vi "UEvent_ON_OFF_POWER_SOURCE.vi"(6 "USB":tag, 7 "Power ON/OFF DUT":enum16{"Power ON DUT", "Power OFF DUT"}(ring), 8 "Ext PW Vol Monitor":bool, 9 "Value":T1, 10 "Vout  - Vbat profile":enum16{"3.8VDC", "2.9VDC", "By Pass", "4.0VDC"}(ring), 11 "Refnum in":refnum<k21>) -> (1 "Battery_Voltage":dbl, 2 "DUT_Voltage":dbl, 3 "Refnum out":refnum<k21>)   [LabVIEW 2015]
uses:
  Range_Shunt_selector.ctl
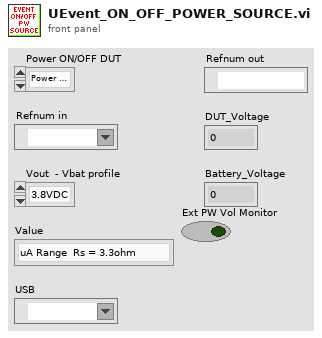
[diagram p1: front panel]
types:
  T1 = typedef "Range_Shunt_selector.ctl" = enum16{"uA Range  Rs = 3.3ohm", "mA Range Rs = 3.3ohm", "mA Range Rs = 1ohm", "mA Range Rs = 1ohm - X2"}
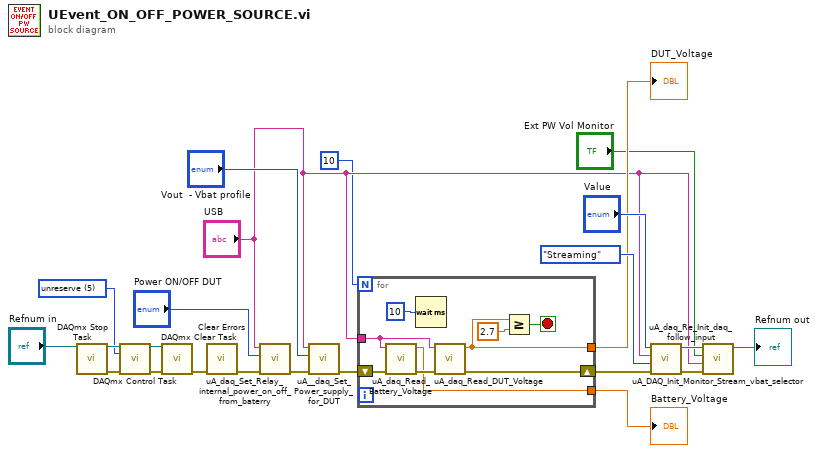
[diagram p0: block diagram]
diagram:
  w1 = 5 items=["verify"=2, "reserve"=4, "commit"=3, "unreserve"=5, "abort"=6] ("action")
  n1 = call <vilib>:"DAQmx Stop Task.vi"("task/channels in"="Refnum in") -> ("task out"=w5:refnum<k21>, "error out"=w3:errorcluster)  [unwired: 13 in]
  n2 = call <vilib>:"DAQmx Control Task.vi"("task/channels in"=w5, "action"=w1, "error in"=w3) -> ("task out"=w4:refnum<k21>, "error out"=w2:errorcluster)  [unwired: 11 in]
  n3 = call <vilib>:"DAQmx Clear Task.vi"("task in"=w4, "error in"=w2) -> ("error out"=w13:errorcluster)  [unwired: 13 in]
  n4 = call <vilib>:"Clear Errors.vi"("error in (no error)"=w13) -> ("error out"=w18:errorcluster)  [unwired: 5 in, 1 out]
  n5 = call "uA_daq_Set_Relay_internal_power_on_off_from_baterry.vi"("error in"=w18, "Power ON/OFF DUT"="Power ON/OFF DUT", "USB DAQ"="USB") -> ("error out"=w20:errorcluster)  [unwired: 8 in]
  n6 = call "uA__daq_Set_Power_supply_for_DUT.vi"("error in"=w20, "DUT Voltage Selector"="Vout  - Vbat profile", "USB DAQ"="USB") -> ("error out"=w7:errorcluster)  [unwired: 8 in]
  n7 = for {
    N: 10 -> [_]
    tunnel: [w26] -> w16
    tunnel: [w30] -> w15
    tunnel: "USB" -> [w29]
    shift-right: [w32] -> w23
    shift-left: w7 -> [w28]
    stop <- w24 stop-if-true
    n8 = call "uA_daq_Read_Battery_Voltage.vi"("error in"=w28, "USB DAQ"=w29) -> ("error out"=w31:errorcluster, "Battery_Voltage"=w30:dbl)  [unwired: 8 in]
    n9 = Wait (ms)(milliseconds to wait=u32 10) -> ()  [unwired: 1 out]
    n10 = call "uA_daq_Read_DUT_Voltage.vi"("error in"=w31, "USB DAQ"=w29) -> ("error out"=w32:errorcluster, "DUT_Voltage"=w26:dbl)  [unwired: 8 in]
    n11 = Greater Or Equal?(x=w26, y=2.7) -> (x >= y?=w24:bool)
  }
  "DUT_Voltage" <- w16
  "Battery_Voltage" <- w15
  n12 = call "uA_daq_Re_Init_daq_follow_input.vi"("error in (no error)"=w23, "Acquire Mode"=enum16{"Streaming", "Read All", "Stop"}."Streaming", "USB"="USB", "Range_shunt"="Value") -> ("error out"=w8:errorcluster, "Refnum out"=w12:refnum<k21>)  [unwired: 6 in]
  n13 = call "uA_DAQ_Init_Monitor_Stream_vbat_selector.vi"("error in (no error)"=w8, "USB"="USB", "Ext PW Vol Monitor"="Ext PW Vol Monitor", "Refnum in"=w12) -> ("Refnum out"=→"Refnum out":refnum<k21>)  [unwired: 6 in, 1 out]
